vi "oa_Concatenate Even Angle Signal and Trigger Indices (N Channels).vi"(7 "reset?":bool, 8 "history trigger indices":T1, 9 "trigger indices":T1, 10 "history even angle signals":cluster{"r0":dbl, "dr":dbl, "Y":dbl[]}[](array[cluster]) {"r0" format="%.2p"; "dr" format="%.2p"; "Y" format="%.2f"}, 11 "even angle signals":cluster{"r0":dbl, "dr":dbl, "Y":dbl[]}[](array[cluster]) {"r0" format="%.2p"; "dr" format="%.2p"; "Y" format="%.2f"}) -> (1 "trigger indices out":T1, 3 "even angle signals out":cluster{"r0":dbl, "dr":dbl, "Y":dbl[]}[](array[cluster]) {"r0" format="%.2p"; "dr" format="%.2p"; "Y" format="%.2f"})   [LabVIEW 2017, in "SoundVib_OAUtility.lvlib"]
uses:
  <vilib>/addons/Sound and Vibration/Order Analysis/Utility/SoundVib_OAUtility.lvlib
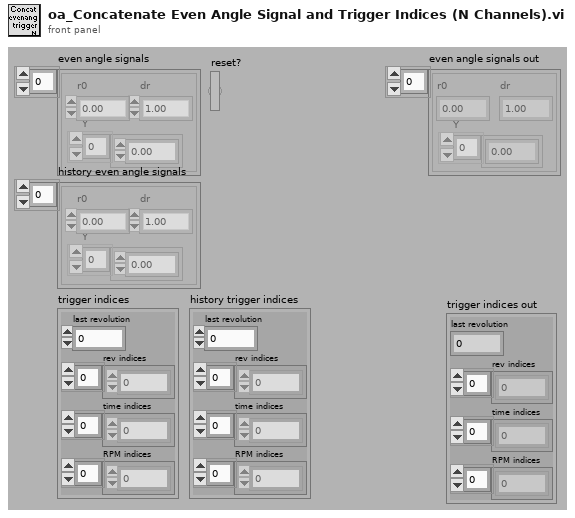
[diagram p1: front panel]
types:
  T1 = cluster{"last revolution":dbl, "rev indices":dbl[], "time indices":dbl[], "RPM indices":dbl[]}
  T2 = cluster{"last revolution":dbl, dbl[], dbl[], dbl[]}
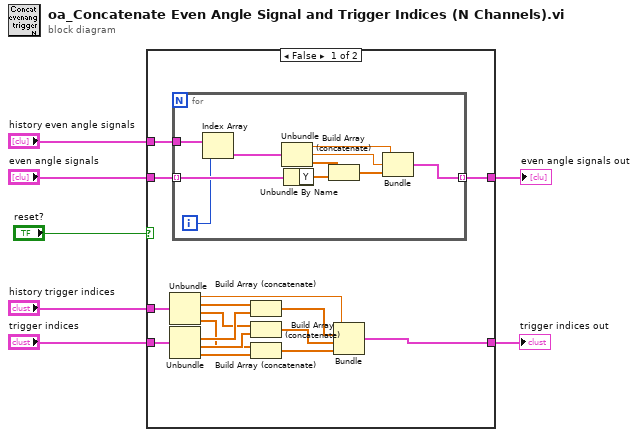
[diagram p0: block diagram]
diagram:
  n1 = case shown="False" "reset?" {
    tunnel: "even angle signals" -> [w23 w35]
    tunnel: [w22 w35] -> w5
    tunnel: "trigger indices" -> [w21 w34]
    tunnel: [w9 w34] -> w3
    tunnel: "history even angle signals" -> [w8 _]
    tunnel: "history trigger indices" -> [w20 _]
    frame False {
      n2 = Unbundle(w20) -> ("last revolution"=w10:dbl, "rev indices"=w19:dbl[], "time indices"=w17:dbl[], "RPM indices"=w15:dbl[])
      n3 = Unbundle(w21) -> ("rev indices"=w18:dbl[], "time indices"=w16:dbl[], "RPM indices"=w14:dbl[])  [unwired: 1 out]
      n4 = for {
        tunnel: w23 -> [w33] mode=indexing
        tunnel: [w27] -> w22 mode=indexing
        tunnel: w8 -> [w26]
        i -> [w24]
        n5 = Index Array(array=w26, index=w24) -> (element=w25:cluster{"r0":dbl, "dr":dbl, "Y":dbl[]})
        n6 = Unbundle(w25) -> ("r0"=w30:dbl, "dr"=w29:dbl, "Y"=w32:dbl[])
        n7 = Unbundle By Name(w33) -> ("Y"=w31:dbl[])
        n8 = Build Array (concatenate)(w32, w31) -> (w28:dbl[])
        n9 = Bundle("r0"=w30, "dr"=w29, w28) -> (w27:cluster{"r0":dbl, "dr":dbl, dbl[]})  [unwired: 1 in]
      }
      n10 = Build Array (concatenate)(w19, w18) -> (w13:dbl[])
      n11 = Build Array (concatenate)(w17, w16) -> (w12:dbl[])
      n12 = Build Array (concatenate)(w15, w14) -> (w11:dbl[])
      n13 = Bundle("last revolution"=w10, w13, w12, w11) -> (w9:T2)  [unwired: 1 in]
    }
    frame True {
    }
  }
  "even angle signals out" <- w5
  "trigger indices out" <- w3
